vi "Write num2.vi"(8 "error in (no error)":errorcluster, 10 "num2":T1, 11 "AbsorbPOrigin in":refnum<class "AbsorbPOrigin.lvclass">) -> (0 "error out":errorcluster, 3 "AbsorbPOrigin out":refnum<class "AbsorbPOrigin.lvclass">)   [LabVIEW 2014, in "TCSDataDefinitions.lvlib" / "TCSCommand.lvlib" / "POriginCommands.lvlib" / "AbsorbPOrigin.lvclass"]
uses:
  AbsorbPOrigin.lvclass
  OffsetCommands/Enumerations/Num2Types.ctl
  AbsorbPOrigin.lvclass/AbsorbPOrigin.ctl
  OffsetCommands/OffsetCommands.lvlib
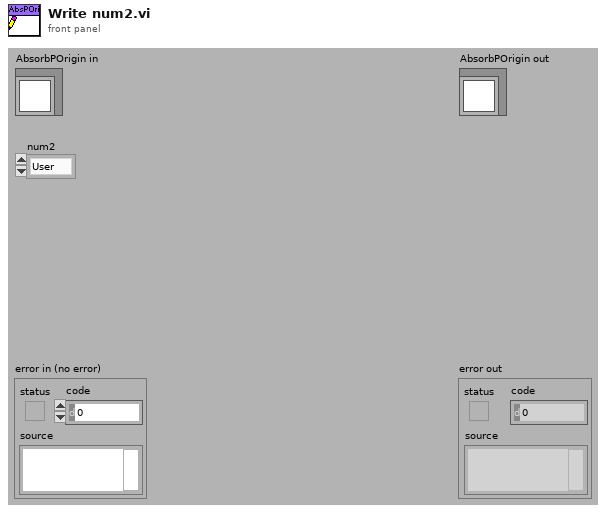
[diagram p1: front panel]
types:
  T1 = typedef "TCSDataDefinitions.lvlib/TCSCommand.lvlib/OffsetCommands.lvlib/Num2Types.ctl" = enum16{"User", "Handset", "Both"}
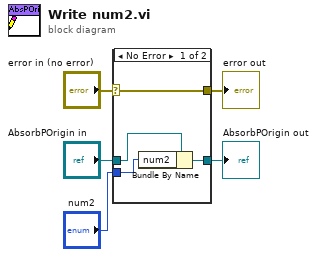
[diagram p0: block diagram]
diagram:
  n1 = case shown="No Error" "error in (no error)" {
    selector: "error in (no error)" -> [w9 w10]
    tunnel: [w9 w10] -> w4
    tunnel: [w7 w11] -> w2
    tunnel: "AbsorbPOrigin in" -> [w8 w11]
    tunnel: "num2" -> [w6 _]
    frame No Error {
      n2 = Bundle By Name(cluster=w8, "num2"=w6) -> (w7:refnum<class "AbsorbPOrigin.lvclass">)
    }
    frame Error {
    }
  }
  "error out" <- w4
  "AbsorbPOrigin out" <- w2
